vi "Release.vi"(8 "error in (no error)":errorcluster, 11 "Scenarios Class in":refnum<class "Scenarios Class.lvclass">) -> (0 "error out":errorcluster)   [LabVIEW 2020, in "SECS Scenarios.lvlib" / "Scenarios Class.lvclass"]
uses:
  Scenarios Class.lvclass
  Scenarios Class.lvclass/Scenarios Class.ctl
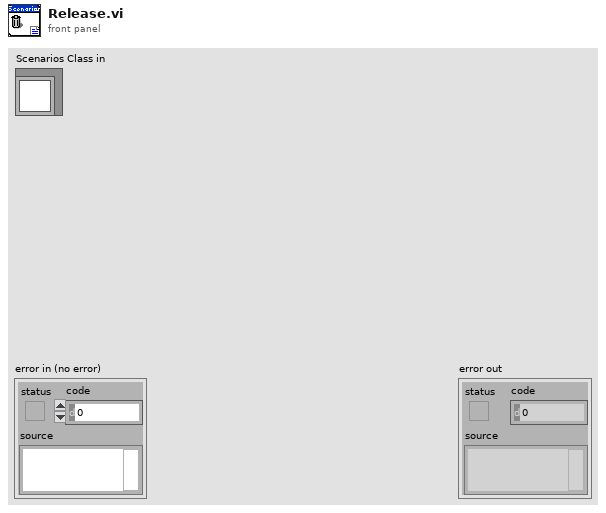
[diagram p1: front panel]
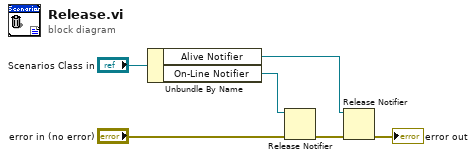
[diagram p0: block diagram]
diagram:
  n1 = Unbundle By Name("Scenarios Class in") -> ("Alive Notifier"=w5:refnum<notifier>, "On-Line Notifier"=w1:refnum<notifier>)
  n2 = Release Notifier(notifier=w1, error in (no error)="error in (no error)") -> (error out=w2:errorcluster)  [unwired: 1 in, 2 out]
  n3 = Release Notifier(notifier=w5, error in (no error)=w2) -> (error out=→"error out":errorcluster)  [unwired: 1 in, 2 out]
